vi "Configure Trigger.vi"(6 "Sample Interval (-1s)":dbl=-1.0 format="%.2f", 7 "Trigger Type Index(0)":u16, 8 "error in (no error)":errorcluster, 9 "Samples per Trigger(1)":i32=1, 10 "Triggers to measure(1)":i32=1, 11 "DMM Driver in":refnum<class "DMM Driver.lvclass">) -> (0 "error out":errorcluster, 1 "Success?":bool, 3 "DMM Driver out":refnum<class "DMM Driver.lvclass">)   [LabVIEW 2020, in "DMM.lvlib" / "DMM Driver.lvclass"]
doc: "Configure the DMM for a triggered measurement.\n\nThe default implementation does nothing."
uses:
  DMM Driver.lvclass
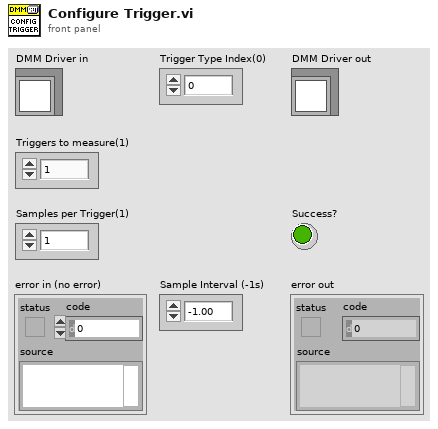
[diagram p1: front panel]
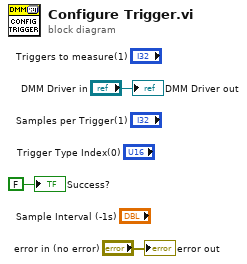
[diagram p0: block diagram]
diagram:
  "error out" <- "error in (no error)"
  "DMM Driver out" <- "DMM Driver in"
  "Success?" <- FALSE ("Success?")
